vi "onDestroy.vi"(8 "error in (no error)":errorcluster, 11 "SMO.InstrumentDriver":refnum<class "SMO.InstrumentDriver.lvclass">) -> (0 "error out":errorcluster, 3 "SMO.InstrumentDriver out":refnum<class "SMO.InstrumentDriver.lvclass">)   [LabVIEW 2013, in "SMO.InstrumentDriver.lvclass"]
doc: "JKI State Machine Objects (SMO) 1.1.4.28\nJKI - JKI\nCopyright (c) 2016, JKI"
uses:
  SMO.InstrumentDriver.lvclass
  <vilib>/JKI/JKI SMO/SMO/SMO.lvclass
panel:
  # "For instructions on how to use the JKI State Machine Objects, examples and video tutorials, visit:\nhttp://jki.net/state-machine-objects/\n\nJKI State Machine Objects™\nhttp://jki.net/state-machine-objects/\nCopyright (C) 2005-2015, JKI <info@jki.net>\nALL RIGHTS RESERVED"
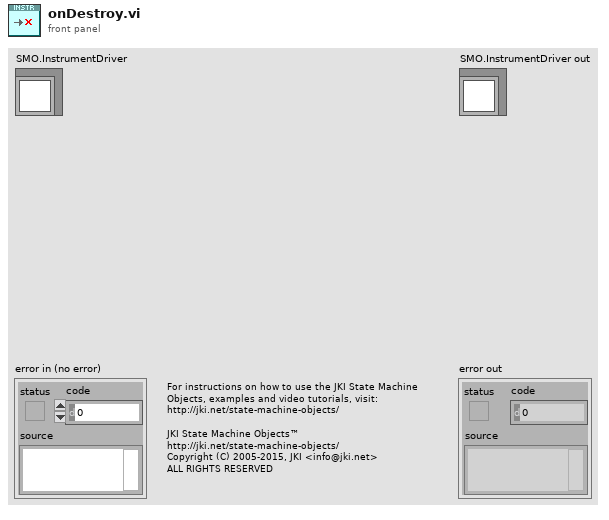
[diagram p1: front panel]
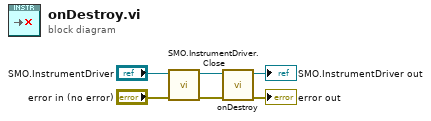
[diagram p0: block diagram]
diagram:
  n1 = call-dynamic "SMO.InstrumentDriver.Close.vi"("error in (no error)"="error in (no error)", "SMO.Instrument"="SMO.InstrumentDriver") -> ("error out"=w1:errorcluster, "SMO.Instrument out"=w3:refnum<class "SMO.InstrumentDriver.lvclass">)  [unwired: 8 in]
  n2 = call-parent "onDestroy.vi"("error in (no error)"=w1, "SMO"=w3) -> ("error out"=→"error out":errorcluster, "SMO out"=→"SMO.InstrumentDriver out":refnum<class "SMO.InstrumentDriver.lvclass">)  [unwired: 8 in]
